vi "set Lexer.vi"(8 "error in (no error)":errorcluster, 10 "Lexer":i32(ring)=15 items=["Container"=0, "Null"=1, "Python"=2, "Cpp"=3, "Html"=4, "Xml"=5, "Perl"=6, "Sql"=7, "Vb"=8, "Properties"=9, "Batch"=12, "Lua"=15, "Pascal"=18, "Ada"=20, "Lisp"=21, "Ruby"=22, "VbScript"=28, "Asm"=34, "Fortran"=36, "Css"=38, "Verilog"=56, "BlitzBasic"=66, "PureBasic"=67, "PhpScript"=69, "Smalltalk"=72, "FreeBasic"=75, "R"=86, "PowerShell"=88, "Markdown"=98, "Json"=120], 11 "ScintillaNET in":refnum<class "ScintillaNET.lvclass">) -> (0 "error out":errorcluster, 3 "ScintillaNET out":refnum<class "ScintillaNET.lvclass">)   [LabVIEW 2018, in "ScintillaNET.lvclass"]
uses:
  ScintillaNET.lvclass
  ScintillaNET.lvclass/ScintillaNET.ctl
  D:/project/hobby/LF2R/LabVIEW/source/ScintillaNET/dll/ScintillaNET.dll
  dll/ScintillaNET.dll
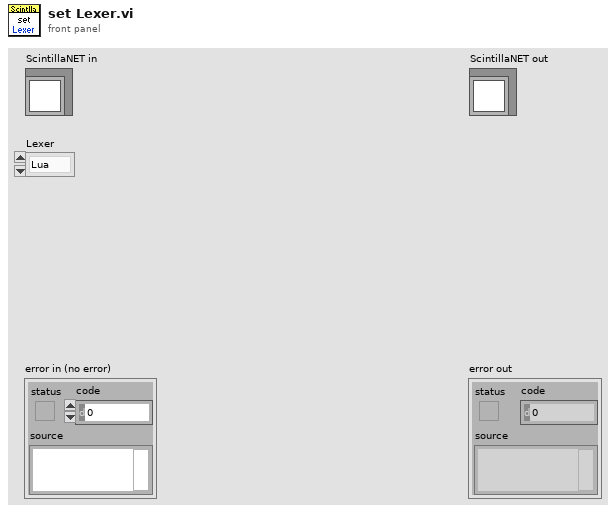
[diagram p1: front panel]
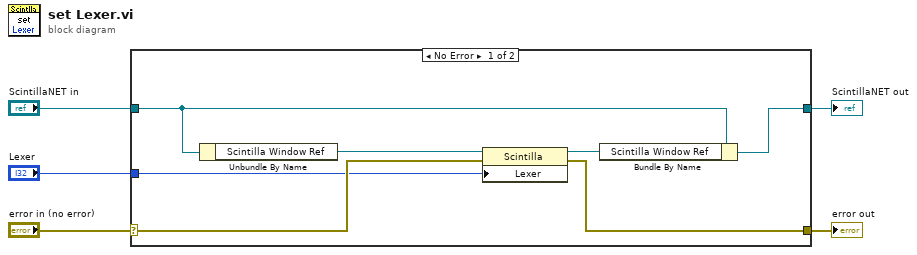
[diagram p0: block diagram]
diagram:
  n1 = case shown="No Error" "error in (no error)" {
    selector: "error in (no error)" -> [w8 w14]
    tunnel: [w7 w14] -> w4
    tunnel: [w11 w13] -> w2
    tunnel: "ScintillaNET in" -> [w12 w13]
    tunnel: "Lexer" -> [w6 _]
    frame No Error {
      n2 = Unbundle By Name(w12) -> ("Scintilla Window Ref"=w10:refnum<k24>)
      n3 = property class="Scintilla"(reference=w10, error in=w8, "Lexer"=w6) -> (reference out=w9:refnum<k24>, error out=w7:errorcluster)
      n4 = Bundle By Name(cluster=w12, "Scintilla Window Ref"=w9) -> (w11:refnum<class "ScintillaNET.lvclass">)
    }
    frame Error {
    }
  }
  "error out" <- w4
  "ScintillaNET out" <- w2
